vi "AB_API Link And Expand.vi"(8 "error in":errorcluster, 11 "Build in":refnum<class "AB_PackedLibrary.lvclass">) -> (0 "error out":errorcluster, 3 "Build out":refnum<class "AB_PackedLibrary.lvclass">)   [LabVIEW 2020]
uses:
  <vilib>/AppBuilder/AB_Classes/PackedLib/AB_PackedLibrary.lvclass
  e:/builds/penguin/labview/branches/2020/dev/dist/vi.lib/AppBuilder/AB_Classes/Build/AB_Build.lvclass
  <vilib>/AppBuilder/AB_Classes/Source/AB_Source.lvclass
  <vilib>/AppBuilder/AB_Classes/Build/AB_Build.lvclass
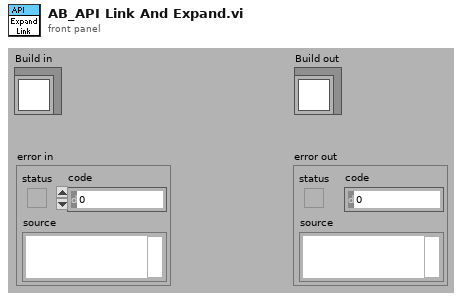
[diagram p1: front panel]
types:
  T1 = typedef "AB_Build.ctl" = cluster{"buildSpecName":string, "buildSpecDescription":string, "destinations":refnum<class "AB_Destination.lvclass">[], "exclusionOption":T2, "defaultLanguage":string, "supportedLanguages":string[], "excludedDirectories":path[], "buildContext":refnum<vi>, "buildObject":T3, "preview":bool, "programatic":bool, "progressBarEvents":T4, "userLog_Path":path, "preActionID":string, "preAction_Path":path, "postActionID":string, "postAction_Path":path, "eng_checkForBrokenVIs?":bool, "eng_verboseLinkerErrors?":bool, "localDest_Path":path, "targetDest_Path":path, "removeVIObject":u16, "cache":refnum<class "PreviewCache.lvclass">, "use cache":bool, "previewCache_ID":string, "buildCache_ID":string, "eng_TempLocalDest_Path":path, "eng_collectDependencies?":bool, "versionInfo":cluster{"buildVersion":cluster{"major":u16, "minor":u16, "patch":u16, "build":u16}, "autoIncrement":bool}, "eng_enableVIChecksums":bool}
  T2 = typedef "AB_Exclusion_Option.ctl" = cluster{"typedefs":bool, "polymorphicVIs":bool, "unusedLibraryItems":bool, "modifyLibraryFile":bool, "edit-timeDependencies":bool, "inlineVIs":bool, "dependent PPLs":bool, "dependent DLLs":bool}
  T3 = typedef "ItemRef.ctl" = u64
  T4 = typedef "provcom_ProgressBar_Events.ctl" = cluster{"newJob":refnum<user-event>, "newItem":refnum<user-event>, "errorMsg":T5, "cancel":refnum<user-event>}
  T5 = typedef "mxLvBuildError.ctl" = refnum<user-event>
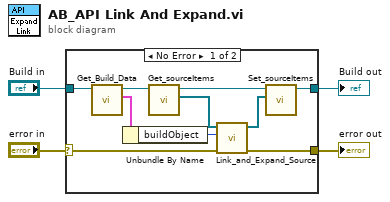
[diagram p0: block diagram]
diagram:
  n1 = case shown="No Error" "error in" {
    selector: "error in" -> [w5 w16]
    tunnel: [w14 w16] -> w4
    tunnel: [w11 w15] -> w3
    tunnel: "Build in" -> [w8 w15]
    frame No Error {
      n2 = call <vilib>:"Get_Build_Data.vi"("Class in"=w8) -> ("data"=w6:T1, "Class out"=w9:refnum<class "AB_PackedLibrary.lvclass">)  [unwired: 8 in, 1 out]
      n3 = Unbundle By Name(w6) -> ("buildObject"=w7:T3)
      n4 = call <vilib>:"Get_sourceItems.vi"("Class in"=w9) -> ("sourceItems"=w12:refnum<class "AB_Source.lvclass">[], "Class out"=w10:refnum<class "AB_PackedLibrary.lvclass">)  [unwired: 8 in, 1 out]
      n5 = call <vilib>:"Link_and_Expand_Source.vi"("error in (no error)"=w5, "Object"=w7, "AB_Source in"=w12) -> ("error out"=w14:errorcluster, "AB_Source out"=w13:refnum<class "AB_Source.lvclass">[])  [unwired: 7 in]
      n6 = call <vilib>:"Set_sourceItems.vi"("sourceItems"=w13, "Class in"=w10) -> ("Class out"=w11:refnum<class "AB_PackedLibrary.lvclass">)  [unwired: 1 in, 8 out]
    }
    frame Error {
    }
  }
  "error out" <- w4
  "Build out" <- w3
